vi "Global dati targa SINUSPENTA.vi"() -> ()   [LabVIEW 2019]
uses:
  SINUS PENTA SANTERNO/controls/Dati targa sinus penta.ctl
panel:
  out "Inverti senso di rotazione KEB":bool
  out "Allarme dati keb":bool
  out "Tempo rampa KEB inviato":bool
  out "Tentativo invio dati KEB":bool
  out "Dati targa KEB Inviati":bool
  out "STATO SINUS":string
  out "Errore Sinus":errorcluster
  in  "T rampa Sinus":dbl
  out "Dati Targa Letti da Sinus":u16[](array[numeric])
  out "Tempo rampa SINUS inviato":bool
  out "Dati targa Sinus Inviati":bool
  in  "T rampa Intesys":dbl
  out "DATI TARGA sinus penta":T1 {"Tensione nominale del motore mot1" format="%.1f"}
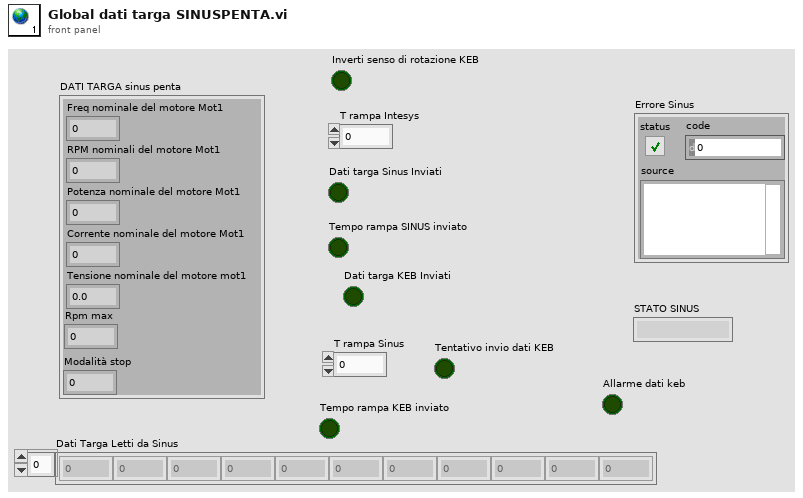
[diagram p1: front panel]
types:
  T1 = typedef "Dati targa sinus penta.ctl" = cluster{"Freq nominale del motore Mot1":dbl, "RPM nominali del motore Mot1":i16, "Potenza nominale del motore Mot1":dbl, "Corrente nominale del motore Mot1":dbl, "Tensione nominale del motore mot1":dbl, "Rpm max":u16, "Modalità stop":u16}
diagram:
